vi "Settings UI.vi"(8 "Show UI":refnum<data-value>, 9 "UI Event Registration":refnum<event-registration>, 11 "Applied Settings":refnum<data-value>) -> ()   [LabVIEW 2020, in "Output Sequencer.lvlib" / "Settings UI.lvclass"]
uses:
  Settings UI.lvclass
  Types/Settings.ctl
  Types/Step Settings.ctl
  Output Sequencer/Types/UI Event.ctl
  Output Sequencer/Types/Event Type.ctl
  Types/Settings UI Action.ctl
  <vilib>/event_ctls.llb/eventvkey.ctl
  Settings UI.lvclass/Settings UI.ctl
  Types/Tree Control Refs.ctl
  Types/Button Refs.ctl
  Types/UI Refs.ctl
  <vilib>/Utility/miscctls.llb/LVPointTypeDef.ctl
  Globals/Dialog Strings.vi
  <vilib>/Platform/browser.llb/Open URL in Default Browser (string).vi
  Output Sequencer/Output Sequencer.lvclass
panel:
  in  "Bottom-Right Tab Control":enum32{"Page 1"}(tab)
  in  "Export":bool
  in  "Apply":bool
  in  "Revert":bool
  in  "Import":bool
  in  "Close":bool
  in  "Remove Step":bool
  in  "Insert Above":bool
  in  "Insert Below":bool
  in  "BottomLeft Tab Control":enum32{"Page 1"}(tab)
  in  "More Info":bool
  out "Setting Description":string
  in  "Expand All":bool
  in  "Collapse All":bool
  in  "Show Overview":bool
  in  "Move Up":bool
  in  "Move Down":bool
  in  "Tab Control":enum32{"Numeric", "String", "Bool", "Enum"}(tab)
  in  "Numeric":dbl min=1.0 max=100.0 step=1.0
  in  "String":string
  in  "Boolean":u16(ring) items=["False", "True"]
  in  "Ring":u16(ring) items=["Disabled", "Enabled"]
  out "Channel Values Preview":waveform(dbl)[](graph)
  in  "Settings Tree":string(tree) caption="Settings"
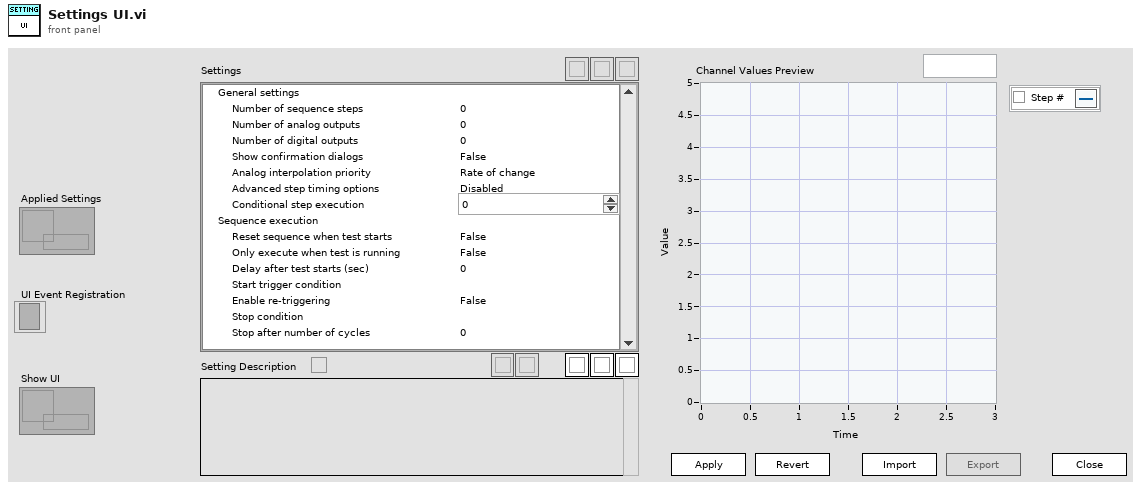
[diagram p1: front panel]
types:
  T1 = typedef "Output Sequencer.lvlib/Settings UI.lvclass/Settings UI Action.ctl" = enum16{"Init", "Timeout", "Tree Change", "Tree Mouse Down/Up", "Value Change", "Expand All", "Show Overview", "Collapse All", "Insert Above", "Insert Below", "Remove Step", "Move Up", "Move Down", "Drag Starting", "Drag Over", "Drop", "Drag Ended", "Import"}
  T2 = typedef "eventvkey.ctl" = enum16{"ASCII", "Enter", "Return", "Shift", "Ctrl", "Alt", "Cmd", "Opt", "Caps", "NumLock", "Clear", "Break", "Up", "Down", "Left", "Right", "Insert", "Delete", "Home", "End", "PageUp", "PageDown", "Escape", "Help", "Pause", "ScrollLock", "F1", "F2", "F3", "F4", "F5", "F6", "F7", "F8", "F9", "F10", "F11", "F12", "F13", "F14", "F15", "F16", "F17", "F18", "F19", "F20", "F21", "F22", "F23", "F24", "Play", "VolumeUp", "VolumeDown", "Mute", "Two Byte Char"}
  T3 = enum32{"Invalid", "Standard", "Closed", "Hidden", "Minimized", "Maximized"}
  T4 = typedef "LVPointTypeDef.ctl" = cluster{"Horizontal":i16, "Vertical":i16}
  T5 = typedef "Output Sequencer.lvlib/Settings UI.lvclass/UI Refs.ctl" = cluster{"Preview Graph":refnum<vi>, "Panel":refnum<vi>, "UI VI":refnum<vi>}
  T6 = typedef "Output Sequencer.lvlib/Settings UI.lvclass/Button Refs.ctl" = cluster{"Apply":refnum<vi>, "Revert":refnum<vi>, "Import":refnum<vi>, "Export":refnum<vi>, "Insert Above":refnum<vi>, "Insert Below":refnum<vi>, "Remove Step":refnum<vi>, "Move Up":refnum<vi>, "Move Down":refnum<vi>}
  T7 = typedef "Output Sequencer.lvlib/Settings UI.lvclass/Tree Control Refs.ctl" = cluster{"Tree Ref":refnum<vi>, "Tab Control":refnum<vi>, "Numeric":refnum<vi>, "String":refnum<vi>, "Boolean":refnum<vi>, "Enum":refnum<vi>, "Tree Item Description":refnum<vi>}
  T8 = typedef "LVPoint32TypeDef.ctl" = cluster{"Horizontal":i32, "Vertical":i32}
  T9 = typedef "Output Sequencer.lvlib/Output Sequencer.lvclass/Event Type.ctl" = enum16{"Channel Update", "Test State Change", "Stop"}
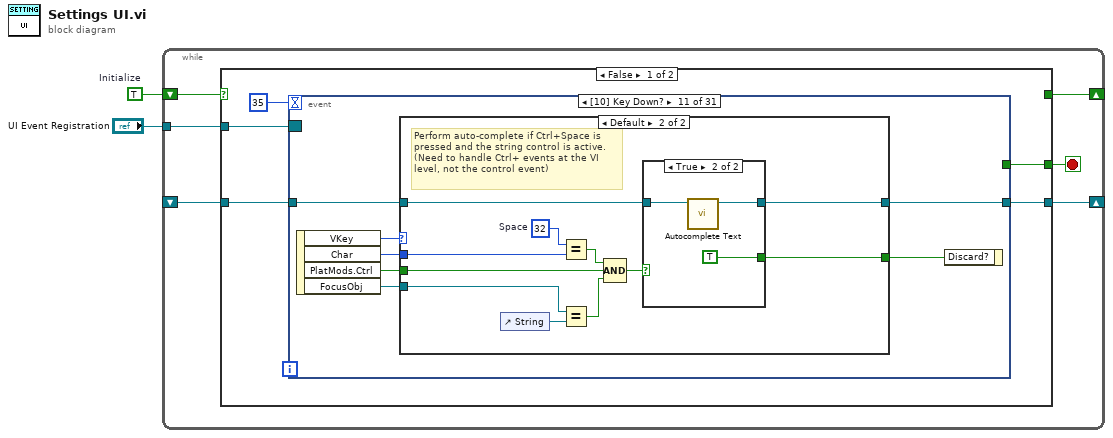
[diagram p0: block diagram]
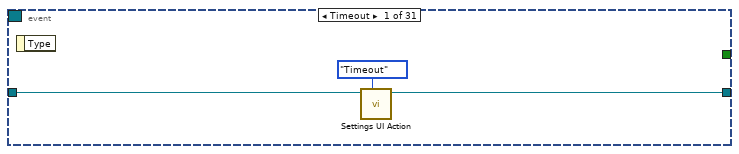
[diagram p2: hidden frame]
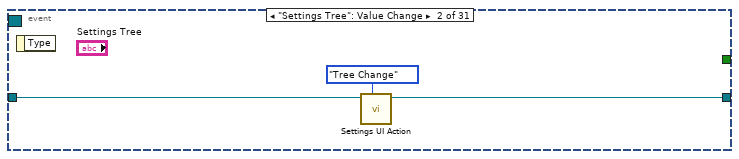
[diagram p3: hidden frame]
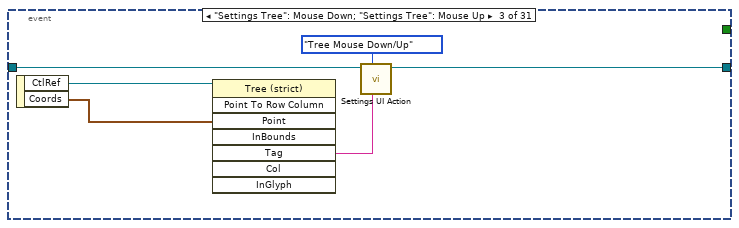
[diagram p4: hidden frame]
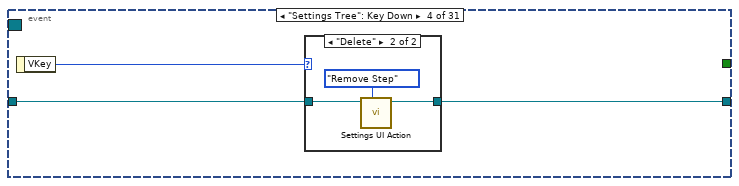
[diagram p5: hidden frame]
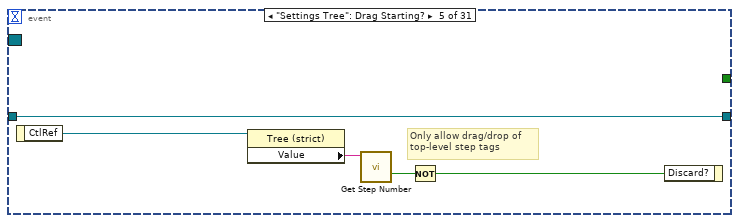
[diagram p7: hidden frame]
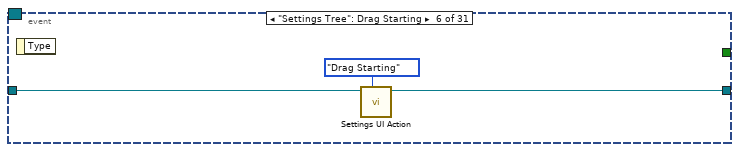
[diagram p8: hidden frame]
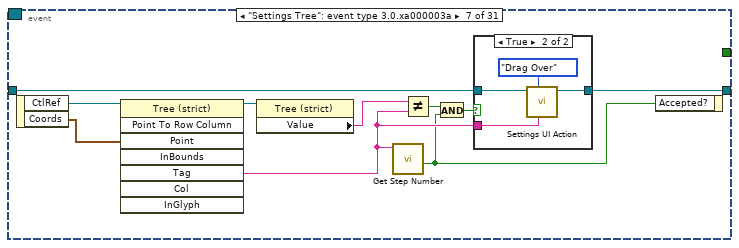
[diagram p9: hidden frame]
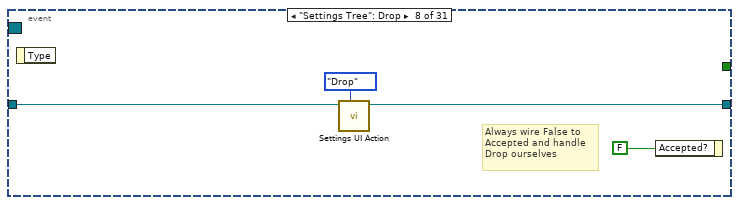
[diagram p11: hidden frame]
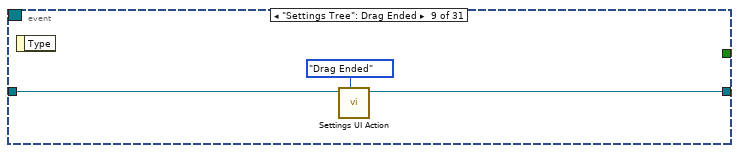
[diagram p12: hidden frame]
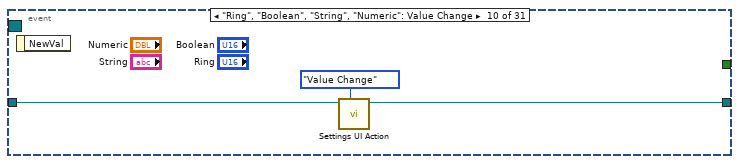
[diagram p13: hidden frame]
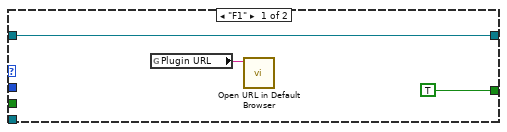
[diagram p14: hidden frame]
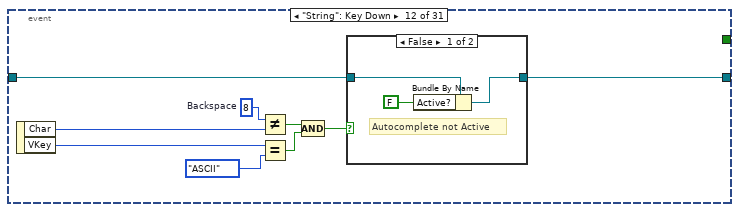
[diagram p16: hidden frame]
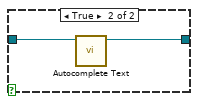
[diagram p17: hidden frame]
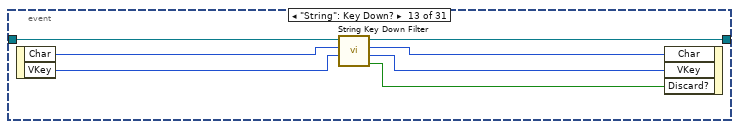
[diagram p18: hidden frame]
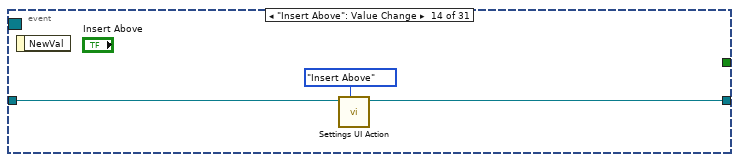
[diagram p19: hidden frame]
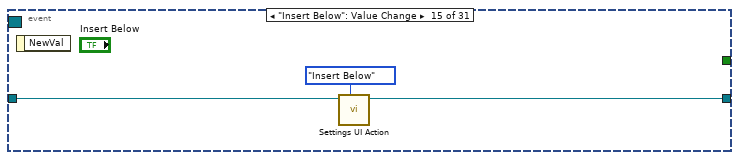
[diagram p20: hidden frame]
diagram:
  w2 = TRUE  # Initialize
  n1 = while {
    tunnel: "UI Event Registration" -> [w8]
    shift-right: [w5] -> _
    shift-left: w2 -> [w6]
    shift-right: [w4] -> _
    shift-left: _ -> [w3]
    stop <- w7 stop-if-true
    n2 = case shown="False" w6 {
      tunnel: w8 -> [w12 _]
      tunnel: [w11 _] -> w7
      tunnel: [_ FALSE] -> w5
      tunnel: [w9 w209] -> w4
      tunnel: w3 -> [w10 _]
      frame False {
        n3 = event shown="[10] Key Down?" {
          selector: w12 -> [_ _ _ _ _ _ _ _ _ _ _ _ _ _ _ _ _ _ _ _ _ _ _ _ _ _ _ _ _ _ _]
          dyn-events: _ -> [_ _ _ _ _ _ _ _ _ _ _ _ _ _ _ _ _ _ _ _ _ _ _ _ _ _ _ _ _ _ _]
          timeout: 35 -> [_ _ _ _ _ _ _ _ _ _ _ _ _ _ _ _ _ _ _ _ _ _ _ _ _ _ _ _ _ _ _]
          tunnel: [_ _ _ _ _ _ _ _ _ _ _ _ _ _ _ _ _ _ _ _ _ _ _ _ _ _ _ _ _ _ w159] -> w11
          tunnel: w10 -> [w16 w18 w21 w27 w33 w39 w43 w57 w61 w64 w69 w92 w109 w113 w116 w119 w122 w124 w127 w130 w133 w136 w139 w140 w144 w146 w148 w149 w153 w155 w157]
          tunnel: [w14 w17 w20 w26 w33 w38 w42 w56 w60 w63 w68 w91 w108 w112 w115 w118 w122 w123 w126 w129 w132 w135 w138 w141 w143 w145 w148 w150 w151 w154 w158] -> w9
          event Timeout {
            n4 = event-data() -> ()  [unwired: 1 in, 1 out]
            n5 = call "Settings UI Action.vi"("Action"=Settings_UI_Action."Timeout" ("Mode"), "UI Data in"=w16) -> ("UI Data out"=w14:refnum<class "Settings UI.lvclass">)  [unwired: 9 in]
          }
          event "Settings Tree": Value Change {
            n6 = event-data() -> ()  [unwired: 1 in, 1 out]
            n7 = call "Settings UI Action.vi"("Action"=Settings_UI_Action."Tree Change" ("Mode"), "UI Data in"=w18) -> ("UI Data out"=w17:refnum<class "Settings UI.lvclass">)  [unwired: 9 in]
          }
          event "Settings Tree": Mouse Down; "Settings Tree": Mouse Up {
            n8 = event-data() -> ("CtlRef"=w24:refnum<vi>, "Coords"=w23:T8)  [unwired: 1 in]
            n9 = invoke on="Invoke Node" class="Tree (strict)" method="Point To Row Column"(reference=w24, "Point"=w23) -> ("Tag"=w22:string)  [unwired: 6 in, 7 out]
            n10 = call "Settings UI Action.vi"("Mouse Interaction Tag"=w22, "Action"=Settings_UI_Action."Tree Mouse Down/Up" ("Mode"), "UI Data in"=w21) -> ("UI Data out"=w20:refnum<class "Settings UI.lvclass">)  [unwired: 8 in]
          }
          event "Settings Tree": Key Down {
            n11 = event-data() -> ("VKey"=w28:T2)  [unwired: 1 in]
            n12 = case shown="\"Delete\"" w28 {
              tunnel: w27 -> [w29 w31]
              tunnel: [w29 w30] -> w26
              frame Default {
              }
              frame "Delete" {
                n13 = call "Settings UI Action.vi"("Action"=Settings_UI_Action."Remove Step" ("Mode"), "UI Data in"=w31) -> ("UI Data out"=w30:refnum<class "Settings UI.lvclass">)  [unwired: 9 in]
              }
            }
          }
          event "Settings Tree": Drag Starting? {
            # "Only allow drag/drop of\ntop-level step tags"
            n14 = event-data() -> ("CtlRef"=w37:refnum<vi>)  [unwired: 1 in]
            n15 = property class="Tree (strict)"(reference=w37) -> ("Value"=w34:string)  [unwired: 1 in, 2 out]
            n16 = call "Get Step Number.vi"("Tree Tag"=w34) -> ("Is Step tag?"=w35:bool)  [unwired: 8 in, 2 out]
            n17 = Not(x=w35) -> (.not. x?=w36:bool)
            n18 = event-data("Discard?"=w36) -> ()  [unwired: 1 in, 1 out]
          }
          event "Settings Tree": Drag Starting {
            n19 = event-data() -> ()  [unwired: 1 in, 1 out]
            n20 = call "Settings UI Action.vi"("Action"=Settings_UI_Action."Drag Starting" ("Mode"), "UI Data in"=w39) -> ("UI Data out"=w38:refnum<class "Settings UI.lvclass">)  [unwired: 9 in]
          }
          event "Settings Tree": event type 3.0.xa000003a {
            n21 = event-data() -> ("CtlRef"=w41:refnum<vi>, "Coords"=w50:T8)  [unwired: 1 in]
            n22 = invoke on="Invoke Node" class="Tree (strict)" method="Point To Row Column"(reference=w41, "Point"=w50) -> (reference out=w49:refnum<vi>, "Tag"=w45:string)  [unwired: 6 in, 6 out]
            n23 = property class="Tree (strict)"(reference=w49) -> ("Value"=w48:string)  [unwired: 1 in, 2 out]
            n24 = call "Get Step Number.vi"("Tree Tag"=w45) -> ("Is Step tag?"=w44:bool)  [unwired: 8 in, 2 out]
            n25 = Not Equal?(x=w48, y=w45) -> (x != y?=w47:bool)
            n26 = And(x=w47, y=w44) -> (x .and. y?=w46:bool)
            n27 = case shown="True" w46 {
              tunnel: w45 -> [_ w54]
              tunnel: w43 -> [w51 w53]
              tunnel: [w51 w52] -> w42
              frame False {
              }
              frame True {
                n28 = call "Settings UI Action.vi"("Mouse Interaction Tag"=w54, "Action"=Settings_UI_Action."Drag Over" ("Mode"), "UI Data in"=w53) -> ("UI Data out"=w52:refnum<class "Settings UI.lvclass">)  [unwired: 8 in]
              }
            }
            n29 = event-data("Accepted?"=w44) -> ()  [unwired: 1 in, 1 out]
          }
          event "Settings Tree": Drop {
            # "Always wire False to\nAccepted and handle\nDrop ourselves"
            n30 = event-data() -> ()  [unwired: 1 in, 1 out]
            n31 = call "Settings UI Action.vi"("Action"=Settings_UI_Action."Drop" ("Mode"), "UI Data in"=w57) -> ("UI Data out"=w56:refnum<class "Settings UI.lvclass">)  [unwired: 9 in]
            n32 = event-data("Accepted?"=FALSE) -> ()  [unwired: 1 in, 1 out]
          }
          event "Settings Tree": Drag Ended {
            n33 = event-data() -> ()  [unwired: 1 in, 1 out]
            n34 = call "Settings UI Action.vi"("Action"=Settings_UI_Action."Drag Ended" ("Mode"), "UI Data in"=w61) -> ("UI Data out"=w60:refnum<class "Settings UI.lvclass">)  [unwired: 9 in]
          }
          event "Ring", "Boolean", "String", "Numeric": Value Change {
            n35 = event-data() -> ()  [unwired: 1 in, 1 out]
            n36 = call "Settings UI Action.vi"("Action"=Settings_UI_Action."Value Change" ("Mode"), "UI Data in"=w64) -> ("UI Data out"=w63:refnum<class "Settings UI.lvclass">)  [unwired: 9 in]
          }
          event Key Down? {
            n37 = event-data() -> ("VKey"=w66:T2, "Char"=w72:i16, "PlatMods.Ctrl"=w71:bool, "FocusObj"=w67:refnum<vi>)  [unwired: 1 in]
            n38 = case shown="Default" w66 {
              tunnel: w72 -> [_ w83]
              tunnel: w71 -> [_ w82]
              tunnel: [TRUE w81] -> w70
              tunnel: w69 -> [w73 w80]
              tunnel: [w73 w79] -> w68
              tunnel: w67 -> [_ w77]
              frame "F1" {
                n39 = global read "Dialog Strings.vi" "Plugin URL"() -> (w75:string)
                n40 = call-poly <vilib>:"Open URL in Default Browser.vi"("URL"=w75) -> ()  [unwired: 5 in, 2 out]
              }
              frame Default {
                w86 = i16 32  # Space
                # "Perform auto-complete if Ctrl+Space is\npressed and the string control is active.\n(Need to handle Ctrl+ events at the VI\nlevel, not the control event)"
                n41 = control-ref of="String"() -> (w78:refnum<vi>)
                n42 = Equal?(x=w86, y=w83) -> (x = y?=w85:bool)
                n43 = Equal?(x=w77, y=w78) -> (x = y?=w76:bool)
                n44 = Compound Arithmetic op=AND(w85, w82, w76) -> (w84:bool)
                n45 = case shown="True" w84 {
                  tunnel: [_ TRUE] -> w81
                  tunnel: w80 -> [w87 w89]
                  tunnel: [w87 w88] -> w79
                  frame False {
                  }
                  frame True {
                    n46 = call "Autocomplete Text.vi"("Settings UI in"=w89) -> ("Settings UI out"=w88:refnum<class "Settings UI.lvclass">)  [unwired: 10 in]
                  }
                }
              }
            }
            n47 = event-data("Discard?"=w70) -> ()  [unwired: 1 in, 1 out]
          }
          event "String": Key Down {
            w97 = i16 8  # Backspace
            n48 = event-data() -> ("Char"=w99:i16, "VKey"=w98:T2)  [unwired: 1 in]
            n49 = Not Equal?(x=w97, y=w99) -> (x != y?=w95:bool)
            n50 = Equal?(x=w98, y=eventvkey."ASCII") -> (x = y?=w94:bool)
            n51 = Compound Arithmetic op=AND(w95, w94) -> (w93:bool)
            n52 = case shown="False" w93 {
              tunnel: [w100 w104] -> w91
              tunnel: w92 -> [w102 w103]
              frame False {
                # "Autocomplete not Active"
                n53 = Bundle By Name(cluster=w102, "Active?"=FALSE) -> (w100:refnum<class "Settings UI.lvclass">)
              }
              frame True {
                n54 = call "Autocomplete Text.vi"("Settings UI in"=w103) -> ("Settings UI out"=w104:refnum<class "Settings UI.lvclass">)  [unwired: 10 in]
              }
            }
          }
          event "String": Key Down? {
            n55 = event-data() -> ("Char"=w111:i16, "VKey"=w110:T2)  [unwired: 1 in]
            n56 = call "String Key Down Filter.vi"("VKey in"=w110, "Char in"=w111, "Settings UI in"=w109) -> ("Discard?"=w107:bool, "VKey out"=w105:T2, "Char out"=w106:i16, "Settings UI out"=w108:refnum<class "Settings UI.lvclass">)  [unwired: 5 in]
            n57 = event-data("Char"=w106, "VKey"=w105, "Discard?"=w107) -> ()  [unwired: 1 in, 1 out]
          }
          event "Insert Above": Value Change {
            n58 = event-data() -> ()  [unwired: 1 in, 1 out]
            n59 = call "Settings UI Action.vi"("Action"=Settings_UI_Action."Insert Above" ("Mode"), "UI Data in"=w113) -> ("UI Data out"=w112:refnum<class "Settings UI.lvclass">)  [unwired: 9 in]
          }
          event "Insert Below": Value Change {
            n60 = event-data() -> ()  [unwired: 1 in, 1 out]
            n61 = call "Settings UI Action.vi"("Action"=Settings_UI_Action."Insert Below" ("Mode"), "UI Data in"=w116) -> ("UI Data out"=w115:refnum<class "Settings UI.lvclass">)  [unwired: 9 in]
          }
          event "Remove Step": Value Change {
            n62 = event-data() -> ()  [unwired: 1 in, 1 out]
            n63 = call "Settings UI Action.vi"("Action"=Settings_UI_Action."Remove Step" ("Mode"), "UI Data in"=w119) -> ("UI Data out"=w118:refnum<class "Settings UI.lvclass">)  [unwired: 9 in]
          }
          event "Channel Values Preview": Plot Attribute Change {
            # "We want the graph to redraw if any plot's visibility changes\nso that the Y-axis autoscales to only the visible plots"
            n64 = event-data() -> ()  [unwired: 1 in, 1 out]
            n65 = Unbundle By Name(w122) -> ("Preview Graph"=w121:refnum<vi>)
            n66 = invoke on="Invoke Node" class="WFGraph (strict)" method="ForceRedraw"(reference=w121) -> ()  [unwired: 2 in, 3 out]
          }
          event "Move Up": Value Change {
            n67 = event-data() -> ()  [unwired: 1 in, 1 out]
            n68 = call "Settings UI Action.vi"("Action"=Settings_UI_Action."Move Up" ("Mode"), "UI Data in"=w124) -> ("UI Data out"=w123:refnum<class "Settings UI.lvclass">)  [unwired: 9 in]
          }
          event "Move Down": Value Change {
            n69 = event-data() -> ()  [unwired: 1 in, 1 out]
            n70 = call "Settings UI Action.vi"("Action"=Settings_UI_Action."Move Down" ("Mode"), "UI Data in"=w127) -> ("UI Data out"=w126:refnum<class "Settings UI.lvclass">)  [unwired: 9 in]
          }
          event "Expand All": Value Change {
            n71 = event-data() -> ()  [unwired: 1 in, 1 out]
            n72 = call "Settings UI Action.vi"("Action"=Settings_UI_Action."Expand All" ("Mode"), "UI Data in"=w130) -> ("UI Data out"=w129:refnum<class "Settings UI.lvclass">)  [unwired: 9 in]
          }
          event "Collapse All": Value Change {
            n73 = event-data() -> ()  [unwired: 1 in, 1 out]
            n74 = call "Settings UI Action.vi"("Action"=Settings_UI_Action."Collapse All" ("Mode"), "UI Data in"=w133) -> ("UI Data out"=w132:refnum<class "Settings UI.lvclass">)  [unwired: 9 in]
          }
          event "Show Overview": Value Change {
            n75 = event-data() -> ()  [unwired: 1 in, 1 out]
            n76 = call "Settings UI Action.vi"("Action"=Settings_UI_Action."Show Overview" ("Mode"), "UI Data in"=w136) -> ("UI Data out"=w135:refnum<class "Settings UI.lvclass">)  [unwired: 9 in]
          }
          event "Apply": Value Change {
            n77 = event-data() -> ()  [unwired: 1 in, 1 out]
            n78 = call "Apply Settings.vi"("Settings UI in"=w139) -> ("Settings UI out"=w138:refnum<class "Settings UI.lvclass">)  [unwired: 10 in]
          }
          event "Revert": Value Change {
            n79 = event-data() -> ()  [unwired: 1 in, 1 out]
            n80 = call "Revert Settings.vi"("Settings UI in"=w140) -> ("Settings UI out"=w141:refnum<class "Settings UI.lvclass">)  [unwired: 10 in]
          }
          event "Import": Value Change {
            n81 = event-data() -> ()  [unwired: 1 in, 1 out]
            n82 = call "Settings UI Action.vi"("Action"=Settings_UI_Action."Import" ("Mode"), "UI Data in"=w144) -> ("UI Data out"=w143:refnum<class "Settings UI.lvclass">)  [unwired: 9 in]
          }
          event "Export": Value Change {
            n83 = event-data() -> ()  [unwired: 1 in, 1 out]
            n84 = call "Export Settings.vi"("Settings UI in"=w146) -> ("Settings UI out"=w145:refnum<class "Settings UI.lvclass">)  [unwired: 10 in]
          }
          event "More Info": Value Change {
            n85 = event-data() -> ()  [unwired: 1 in, 1 out]
            n86 = global read "Dialog Strings.vi" "Plugin URL"() -> (w147:string)
            n87 = call-poly <vilib>:"Open URL in Default Browser.vi"("URL"=w147) -> ()  [unwired: 5 in, 2 out]
          }
          event "Close": Value Change {
            n88 = event-data() -> ()  [unwired: 1 in, 1 out]
            n89 = call "Close UI.vi"("Settings UI in"=w149) -> ("Settings UI out"=w150:refnum<class "Settings UI.lvclass">)  [unwired: 10 in]
          }
          event Panel Resize {
            n90 = event-data() -> ()  [unwired: 1 in, 1 out]
            n91 = call "Update Graph Legend.vi"("UI Data in"=w153) -> ("UI Data out"=w152:refnum<class "Settings UI.lvclass">)  [unwired: 10 in]
            n92 = call "Update Tree Height.vi"("Settings UI in"=w152) -> ("Settings UI out"=w151:refnum<class "Settings UI.lvclass">)  [unwired: 10 in]
          }
          event Panel Close? {
            n93 = event-data() -> ()  [unwired: 1 in, 1 out]
            n94 = call "Close UI.vi"("Settings UI in"=w155) -> ("Settings UI out"=w154:refnum<class "Settings UI.lvclass">)  [unwired: 10 in]
            n95 = event-data("Discard?"=TRUE) -> ()  [unwired: 1 in, 1 out]
          }
          event User Event {
            n96 = event-data() -> ("UsrEvtRef"=w161:refnum<user-event>, "Type"=w162:T9, "Data"=w160:variant)  [unwired: 1 in]
            n97 = case shown="\"Channel Update\"" w162 {
              tunnel: w161 -> [_ _ _ w177]
              tunnel: w160 -> [_ w168 w173 _]
              tunnel: [_ _ _ TRUE] -> w159
              tunnel: [w163 w164 w170 w174] -> w158
              tunnel: w157 -> [w163 w166 w171 w174]
              frame Default {
              }
              frame "Channel Update" {
                n98 = Variant To Data(type=string[] [], Variant=w168) -> (data=w165:string[])  [unwired: 1 in, 1 out]
                n99 = Bundle By Name(cluster=w166, "Mapped Channels"=w165) -> (w164:refnum<class "Settings UI.lvclass">)
              }
              frame "Test State Change" {
                w172 = FALSE  # Test in Progress
                n100 = Variant To Data(type=w172, Variant=w173) -> (data=w169:bool)  [unwired: 1 in, 1 out]
                n101 = call "Test State Change.vi"("Test in Progress"=w169, "Settings UI in"=w171) -> ("Settings UI out"=w170:refnum<class "Settings UI.lvclass">)  [unwired: 9 in]
              }
              frame "Stop" {
                n102 = Destroy User Event(user event=w177) -> ()  [unwired: 1 in, 1 out]
                n103 = property class="VI"("FP.State"=T3."Closed" ("Front Panel Window:State")) -> ()  [unwired: 2 in, 2 out]
              }
            }
          }
        }
      }
      frame True {
        n104 = control-ref of="This VI"() -> (w212:refnum<vi>)
        n105 = control-ref of="Channel Values Preview"() -> (w188:refnum<vi>)
        n106 = control-ref of="Settings Tree"() -> (w206:refnum<vi>)
        n107 = control-ref of="Tab Control"() -> (w205:refnum<vi>)
        n108 = property class="VI"(reference=w212) -> (reference out=w178:refnum<vi>, "Panel"=w187:refnum<vi>)  [unwired: 1 in, 1 out]
        n109 = control-ref of="Numeric"() -> (w204:refnum<vi>)
        n110 = control-ref of="String"() -> (w203:refnum<vi>)
        n111 = control-ref of="Setting Description"() -> (w200:refnum<vi>)
        n112 = control-ref of="Boolean"() -> (w202:refnum<vi>)
        n113 = control-ref of="Ring"() -> (w201:refnum<vi>)
        n114 = Bundle(cluster=T5 {"Preview Graph"=refnum, "Panel"=refnum, "UI VI"=refnum} ("UI Refs"), "Preview Graph"=w188, "Panel"=w187, "UI VI"=w178) -> (w186:T5)
        n115 = Bundle(cluster=T7 {"Tree Ref"=refnum, "Tab Control"=refnum, "Numeric"=refnum, "String"=refnum, "Boolean"=refnum, "Enum"=refnum, "Tree Item Description"=refnum} ("Tree Control Refs"), "Tree Ref"=w206, "Tab Control"=w205, "Numeric"=w204, "String"=w203, "Boolean"=w202, "Enum"=w201, "Tree Item Description"=w200) -> (w184:T7)
        n116 = control-ref of="Apply"() -> (w198:refnum<vi>)
        n117 = control-ref of="Revert"() -> (w197:refnum<vi>)
        n118 = control-ref of="Import"() -> (w196:refnum<vi>)
        n119 = control-ref of="Export"() -> (w195:refnum<vi>)
        n120 = control-ref of="Insert Above"() -> (w194:refnum<vi>)
        n121 = control-ref of="Insert Below"() -> (w193:refnum<vi>)
        n122 = control-ref of="Remove Step"() -> (w192:refnum<vi>)
        n123 = control-ref of="Move Up"() -> (w191:refnum<vi>)
        n124 = control-ref of="Move Down"() -> (w190:refnum<vi>)
        n125 = Bundle(cluster=T6 {"Apply"=refnum, "Revert"=refnum, "Import"=refnum, "Export"=refnum, "Insert Above"=refnum, "Insert Below"=refnum, "Remove Step"=refnum, "Move Up"=refnum, "Move Down"=refnum} ("Button Refs"), "Apply"=w198, "Revert"=w197, "Import"=w196, "Export"=w195, "Insert Above"=w194, "Insert Below"=w193, "Remove Step"=w192, "Move Up"=w191, "Move Down"=w190) -> (w185:T6)
        n126 = property class="Pnl"(reference=w187) -> ("Panes[]"=w181:refnum<vi>[])  [unwired: 1 in, 2 out]
        n127 = Index Array(array=w181) -> (element=w180:refnum<vi>)  [unwired: 1 in]
        n128 = Bundle By Name(cluster=refnum<class "Settings UI.lvclass"> refnum ("Sequencer with Output Values.lvlib:Sequencer Settings.lvclass"), "Tree Control Refs"=w184, "Button Refs"=w185, "UI Refs"=w186, "Show UI ref"="Show UI", "Applied Settings ref"="Applied Settings") -> (w208:refnum<class "Settings UI.lvclass">)
        n129 = property class="Pane"(reference=w180, "Origin"=T4 {"Horizontal"=0, "Vertical"=0}) -> ()  [unwired: 1 in, 2 out]
        n130 = call "Settings UI Action.vi"("Action"=Settings_UI_Action."Init" ("Mode"), "UI Data in"=w208) -> ("UI Data out"=w209:refnum<class "Settings UI.lvclass">)  [unwired: 9 in]
      }
    }
  }
